vi "Get configuration chain.vi"(8 "error in (no error)":errorcluster, 11 "ChatBase in":refnum<class "Chat.lvclass">) -> (0 "error out":errorcluster, 1 "class name":string[](array[string]), 2 "configuration chain":variant[](array[variant]), 3 "ChatBase out":refnum<class "Chat.lvclass">)   [LabVIEW 2012, in "Chat.lvclass"]
doc: "Returns an array of variants containing the configuration clusters of each class in the inheritance chain (lowest child class first), together with an array of all class names in the inheritance chain.\n\nFor classes without configuration cluster, the configuration chain contains empty variants."
uses:
  Chat.lvclass
  <vilib>/Distrio/Murmex/Murmex/Murmex.lvclass
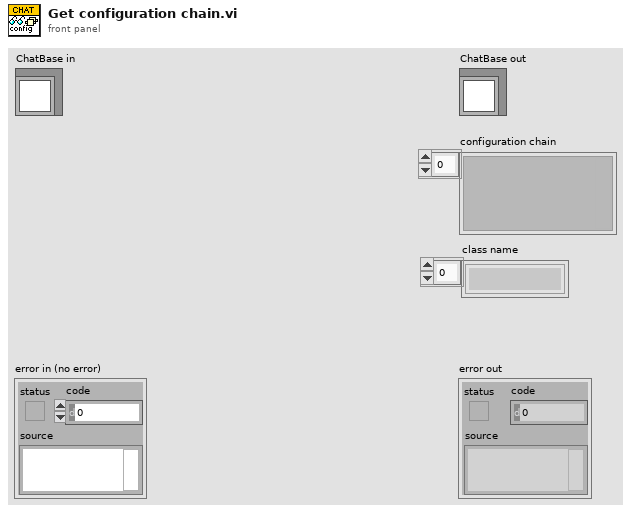
[diagram p1: front panel]
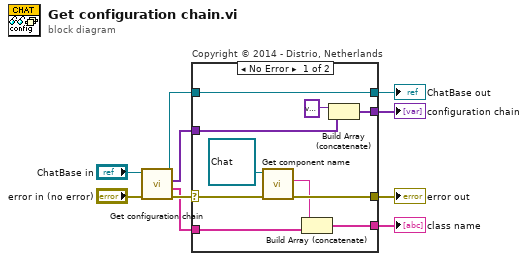
[diagram p0: block diagram]
diagram:
  n1 = call-parent "Get configuration chain.vi"("error in (no error)"="error in (no error)", "MurmexBase in"="ChatBase in") -> ("error out"=w8:errorcluster, "class name"=w5:string[], "configuration chain"=w6:variant[], "MurmexBase out"=w7:refnum<class "Chat.lvclass">)  [unwired: 6 in]
  n2 = case "Copyright © 2014 - Distrio, Netherlands" shown="No Error" w8 {
    selector: w8 -> [w20 w22]
    tunnel: [w19 w22] -> w4
    tunnel: [w14 w21] -> w1
    tunnel: w7 -> [w14 w21]
    tunnel: [w17 _] -> w3
    tunnel: [w16 _] -> w2
    tunnel: w6 -> [w12 _]
    tunnel: w5 -> [w11 _]
    frame No Error {
      n3 = call <vilib>:"Get component name.vi"("error in (no error)"=w20, "Murmex in"=refnum<class "Chat.lvclass"> refnum ("Chat.lvclass")) -> ("error out"=w19:errorcluster, "component name"=w18:string)  [unwired: 7 in, 1 out]
      n4 = Build Array (concatenate)(w18, w11) -> (w17:string[])
      n5 = Build Array (concatenate)(variant ("variant"), w12) -> (w16:variant[])
    }
    frame Error {
    }
  }
  "error out" <- w4
  "ChatBase out" <- w1
  "configuration chain" <- w2
  "class name" <- w3
